vi "Global anno.vi"() -> ()   [LabVIEW 2019]
panel:
  in  "anno":string
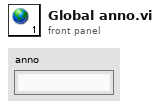
[diagram p1: front panel]
diagram:
